vi "Index 3D Array (returns 1D Array).vi"(10 "index":i32, 11 "3D array":dbl[][][](array[numeric])) -> (3 "1D array":dbl[](array[numeric]))   [LabVIEW 2014]
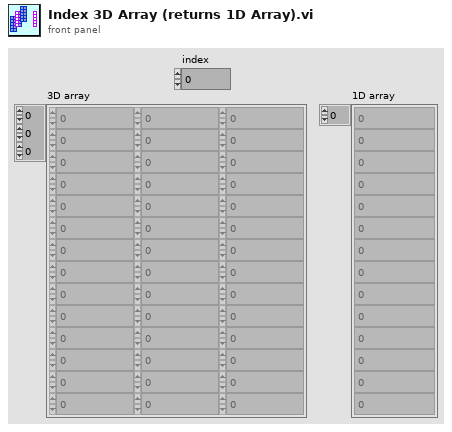
[diagram p1: front panel]
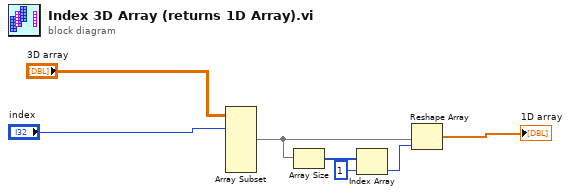
[diagram p0: block diagram]
diagram:
  n1 = Array Subset(array="3D array", index (dim 0)="index") -> (w1:dbl[][][])  [unwired: 5 in]
  n2 = Array Size(array=w1) -> (size(s)=w2:i32[])
  n3 = Index Array(array=w2, index=1) -> (element=w4:i32)
  n4 = Reshape Array(w1, w4) -> (→"1D array":dbl[])
